vi "Sine-squared ramp.vi"(5 "samples":i32=8) -> (0 "error":i32, 1 "sine^2 Ramp":dbl[](array[numeric])=[0.0, 0.002451791281132127, 0.035439982326093925, 0.15111842453404034, 0.3736393584903548, 0.6589297841848273, 0.9034206591835512, 1.0] format="%.4f")   [LabVIEW 2020]
doc: "Generates an array containing a ramp pattern."
uses:
  <vilib>/Analysis/NI_AALBase.lvlib
panel:
  # "sine squared Ramp"
  # "`"
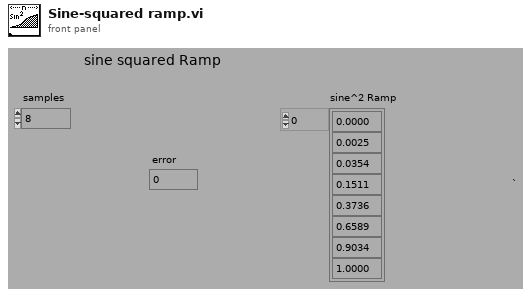
[diagram p1: front panel]
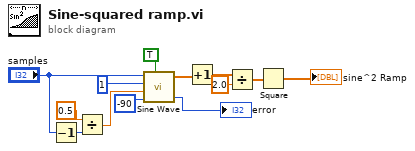
[diagram p0: block diagram]
diagram:
  n1 = Decrement(x="samples") -> (x-1=w8:i32)
  n2 = Divide(x=0.5, y=w8) -> (x/y=w12:dbl)
  n3 = call <vilib>:"Sine Wave.vi"("samples"="samples", "amplitude"=1, "frequency"=w12, "phase in"=-90, "reset phase"=TRUE) -> ("sine wave"=w5:dbl[], "error"=→"error":i32)  [unwired: 1 out]
  n4 = Increment(x=w5) -> (x+1=w4:dbl[])
  n5 = Divide(x=w4, y=2.0) -> (x/y=w2:dbl[])
  n6 = Square(x=w2) -> (x^2=→"sine^2 Ramp":dbl[])
